vi "M-227 Stage Engine.vi"(0 "Unique Notifier Name":string="LevelStage", 11 "COM Port":string[](array[string])) -> ()   [LabVIEW 2016]
uses:
  Stages Controls/Stage Focus Control.ctl
  Stages Controls/Stage Status.ctl
  Stages Controls/Stage Notifier Element.ctl
  Stages Controls/Stage Actions.ctl
  <vilib>/Instr/_visa.llb/VISA Configure Serial Port (Instr).vi
panel:
  out "Position":dbl[](array[numeric])
  in  "Axis":T1={"Axis 1"=TRUE, "Axis 2"=TRUE, "Axis 3"=TRUE}
  in  "ReInitialize":bool
  in  "Abort":bool
  in  "Velocity":dbl(ring)=0.05 items=["SUPER SLOW"=0.01, "SLOW"=0.05, "MEDIUM"=0.1, "FAST"=0.8]
  out "Status":T2
  in  "QUIT":bool
  in  "Focus Control":T3
  # "Left near"
  # "Left far"
  # "Right"
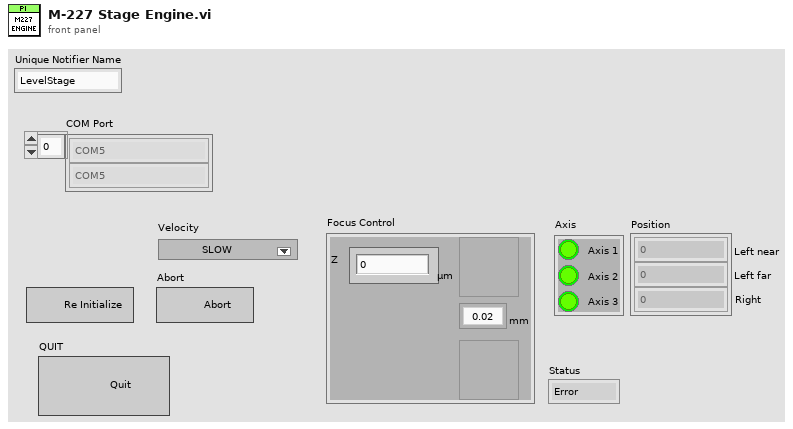
[diagram p1: front panel]
types:
  T1 = cluster{"Axis 1":bool, "Axis 2":bool, "Axis 3":bool}
  T2 = typedef "Stage Status.ctl" = enum16{"Error", "Abort", "Busy", "On Target"}
  T3 = typedef "Stage Focus Control.ctl" = cluster{"Focus Step (um)":enum16{"0.02", "0.05", "0.1", "0.5", "1", "2", "5", "10", "20"}, "Focus Up":bool, "Focus Down":bool, "Z ":dbl}
  T4 = typedef "Stage Actions.ctl" = enum16{"Get Position", "MVR", "MOVE", "HALT", "ONTARGET", "ERROR", "REFERENCE", "INIT", "VELOCITY", "STATUS", "EXIT", "HOME", "ZEROPOS", "NANOPOS", "ANALOG", "QUIT"}
  T5 = typedef "Stage Notifier Element.ctl" = cluster{"Action":T4, "Axis":bool[], "Setpoint":dbl[], "Velocity":dbl, "Cmd Recvd?":bool, "Position":dbl[], "Status":T2, "Misc":variant}
  T6 = cluster{"Focus Step (um)":bool, "Focus Up":bool, "Focus Down":bool, "Z ":bool}
  T7 = enum16{"0.02", "0.05", "0.1", "0.5", "1", "2", "5", "10", "20"}
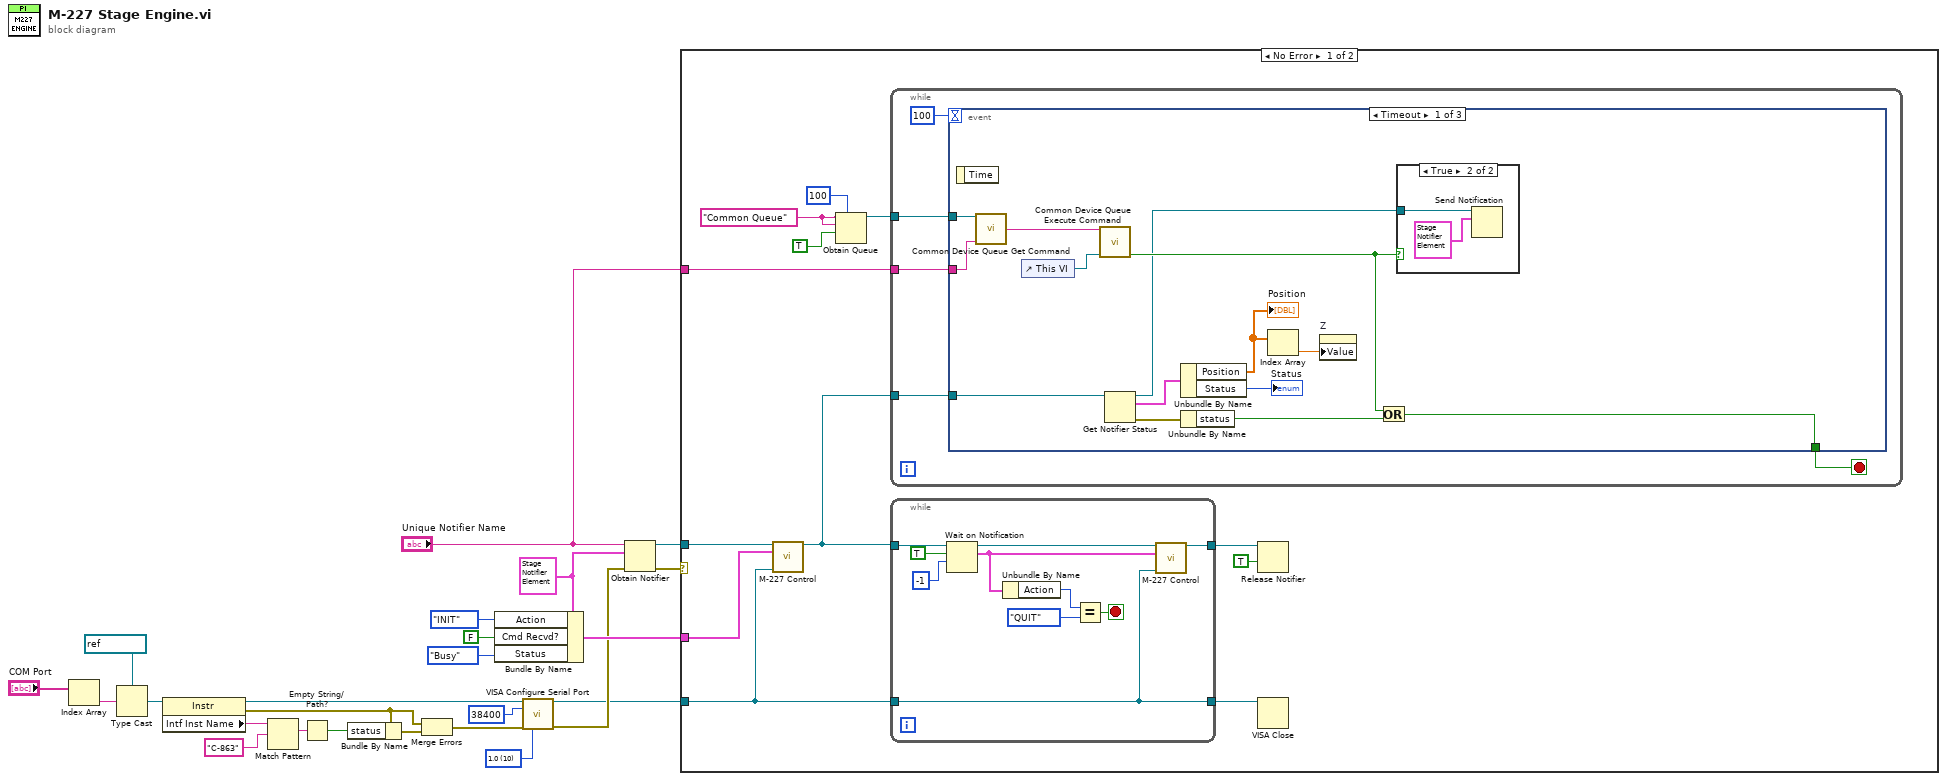
[diagram p0: block diagram]
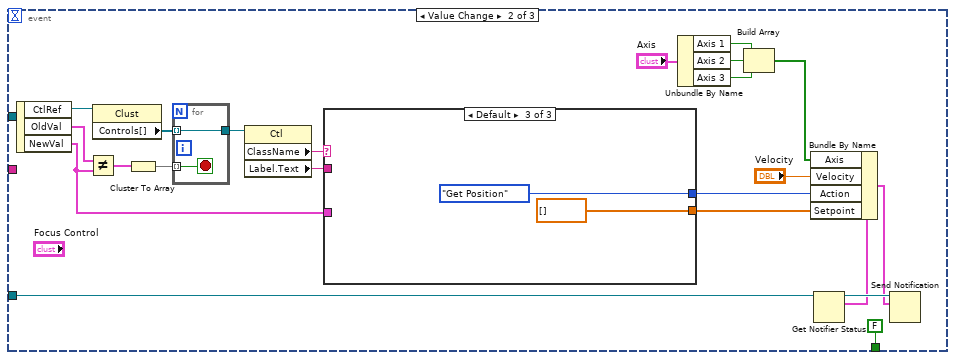
[diagram p3: hidden frame]
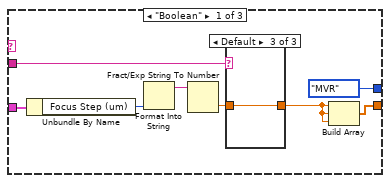
[diagram p4: hidden frame]
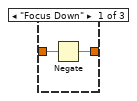
[diagram p5: hidden frame]
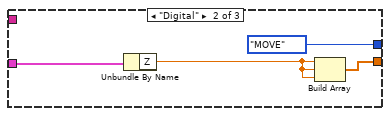
[diagram p7: hidden frame]
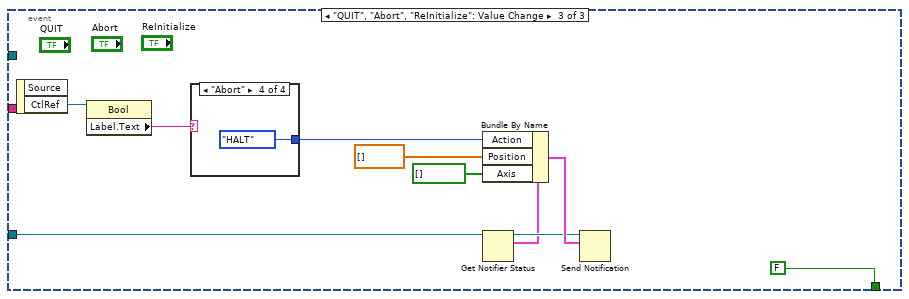
[diagram p8: hidden frame]
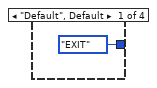
[diagram p9: hidden frame]
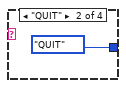
[diagram p10: hidden frame]
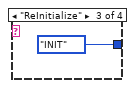
[diagram p11: hidden frame]
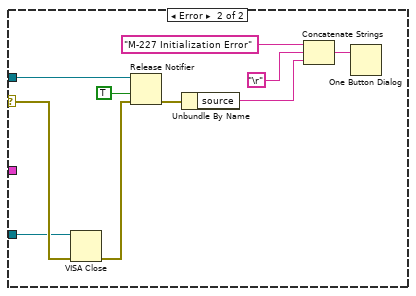
[diagram p12: hidden frame]
diagram:
  w7 = u16 10 items=["1.0"=10, "1.5"=15, "2.0"=20] ("stop bits (10: 1 bit)")
  w11 = T5 {"Action"=enum."Get Position", "Axis"=[], "Setpoint"=[], "Velocity"=0.5, "Cmd Recvd?"=FALSE, "Position"=[], "Status"=enum."Abort", "Misc"=variant} ("Stage Status")
  n1 = Index Array(array="COM Port") -> (element=w17:string)  [unwired: 1 in]
  n2 = Type Cast(type=refnum<visa-resource-name> "COM5" ("reference out"), x=w17) -> (*(type *) &x=w15:refnum<visa-resource-name>)
  n3 = property class="Instr"(reference=w15) -> (reference out=w4:refnum<visa-resource-name>, error out=w20:errorcluster, "Intf Inst Name"=w22:string)  [unwired: 1 in]
  n4 = Match Pattern(string=w22, regular expression="C-863") -> (match substring=w24:string)  [unwired: 1 in, 3 out]
  n5 = Empty String/Path?(string/path=w24) -> (empty?=w21:bool)
  n6 = Bundle By Name(cluster=w20, "status"=w21) -> (w19:errorcluster)
  n7 = Merge Errors(w20, w19) -> (w3:errorcluster)
  n8 = Bundle By Name(cluster=w11, "Action"=Stage_Actions."INIT", "Cmd Recvd?"=FALSE, "Status"=Stage_Status."Busy") -> (w9:T5)
  n9 = call-poly "VISA Configure Serial Port"("VISA resource name"=w4, "baud rate (9600)"=u32 38400, "error in (no error)"=w3, "stop bits (10: 1 bit)"=w7) -> ("VISA resource name out"=w2:refnum<visa-resource-name>, "error out"=w6:errorcluster)  [unwired: 10 in]
  n10 = Obtain Notifier(name (unnamed)="Unique Notifier Name", notification data type=w11, error in (no error)=w6) -> (notifier out=w1:refnum<notifier>, error out=w10:errorcluster)  [unwired: 1 in, 1 out]
  n11 = case shown="No Error" w10 {
    selector: w10 -> [_ w125]
    tunnel: w2 -> [w27 w124]
    tunnel: w9 -> [w28 _]
    tunnel: "Unique Notifier Name" -> [w31 _]
    tunnel: w1 -> [w30 w126]
    frame No Error {
      w33 = "Common Queue" ("Unique Notifier Name")
      n12 = call "M-227 Control.vi"("M-227 Notifier"=w30, "Stage Action"=w28, "VISA In"=w27) -> ("M-227 Notifier (Dup)"=w29:refnum<notifier>)  [unwired: 12 in]
      n13 = Obtain Queue(max queue size (-1, unlimited)=100, name (unnamed)=w33, element data type=w33, create if not found? (T)=TRUE) -> (queue out=w32:refnum<queue>)  [unwired: 1 in, 2 out]
      n14 = while {
        tunnel: w29 -> [w49]
        tunnel: w32 -> [w48]
        tunnel: w31 -> [w47]
        stop <- w50 stop-if-true
        n15 = event shown="[0] Timeout" {
          selector: _ -> [_ _ _]
          dyn-events: _ -> [_ _ _]
          timeout: 100 -> [_ _ _]
          tunnel: [w54 FALSE ("status") FALSE ("status")] -> w50
          tunnel: w49 -> [w64 w78 w115]
          tunnel: w48 -> [w57 _ _]
          tunnel: w47 -> [w56 _ _]
          event Timeout {
            n16 = event-data() -> ()  [unwired: 1 in, 1 out]
            n17 = call "Common Device Queue Get Command.vi"("Common Queue"=w57, "Notifier Name"=w56) -> ("Command"=w59:string)  [unwired: 12 in, 1 out]
            n18 = control-ref of="This VI"() -> (w58:refnum<vi>)
            n19 = call "Common Device Queue Execute Command.vi"("Common Command"=w59, "VI Refnum"=w58) -> ("Quit?"=w53:bool)  [unwired: 12 in, 1 out]
            n20 = Get Notifier Status(notifier=w64) -> (notifier out=w52:refnum<notifier>, current notification=w63:T5, error out=w61:errorcluster)  [unwired: 1 in, 2 out]
            n21 = Unbundle By Name(w63) -> ("Position"=w62:dbl[], "Status"=→"Status":T2)
            "Position" <- w62
            n22 = Unbundle By Name(w61) -> ("status"=w55:bool)
            n23 = Index Array(array=w62) -> (element=w65:dbl)  [unwired: 1 in]
            n24 = property on="Z" class="DigNum (strict)"("Value"=w65) -> ()  [unwired: 2 in, 2 out]
            n25 = Or(x=w53, y=w55) -> (x .or. y?=w54:bool)
            n26 = case shown="True" w53 {
              tunnel: w52 -> [_ w67]
              frame False {
              }
              frame True {
                n27 = Send Notification(notification=T5 {"Action"=enum."QUIT", "Axis"=[], "Setpoint"=[], "Velocity"=0.5, "Cmd Recvd?"=FALSE, "Position"=[], "Status"=enum."Error", "Misc"=variant} ("Stage Status"), notifier=w67) -> ()  [unwired: 1 in, 2 out]
              }
            }
          }
          event Value Change {
            n28 = event-data() -> ("CtlRef"=w88:refnum<vi>, "OldVal"=w89:T3, "NewVal"=w82:T3)  [unwired: 1 in]
            n29 = Not Equal?(x=w89, y=w82) -> (x != y?=w87:T6)
            n30 = property class="Clust"(reference=w88) -> ("Controls[]"=w85:refnum<vi>[])  [unwired: 1 in, 2 out]
            n31 = Cluster To Array(cluster=w87) -> (array=w86:bool[])
            n32 = for {
              tunnel: w86 -> [w109] mode=indexing
              tunnel: [w108] -> w84
              tunnel: w85 -> [w108] mode=indexing
              stop <- w109 stop-if-true
            }
            n33 = property class="Ctl"(reference=w84) -> ("ClassName"=w83:string, "Label.Text"=w81:string)  [unwired: 1 in, 2 out]
            n34 = case shown="Default" w83 {
              tunnel: w82 -> [w96 w105 _]
              tunnel: w81 -> [w97 _ _]
              tunnel: [w92 w104 dbl[] []] -> w80
              tunnel: [Stage_Actions."MVR" ("Action") Stage_Actions."MOVE" ("Action") Stage_Actions."Get Position" ("Action")] -> w77
              frame "Boolean" {
                n35 = Unbundle By Name(w96) -> ("Focus Step (um)"=w94:T7)
                n36 = Format Into String(w94) -> (resulting string=w95:string)  [unwired: 3 in, 1 out]
                n37 = Fract/Exp String To Number(string=w95) -> (number=w93:dbl)  [unwired: 3 in, 1 out]
                n38 = case shown="Default" w97 {
                  tunnel: w93 -> [w99 w100 w101]
                  tunnel: [w98 w100 w101] -> w90
                  frame "Focus Down" {
                    n39 = Negate(x=w99) -> (-x=w98:dbl)
                  }
                  frame "Focus Up" {
                  }
                  frame Default {
                  }
                }
                n40 = Build Array(w90, w90, w90) -> (w92:dbl[])
              }
              frame "Digital" {
                n41 = Unbundle By Name(w105) -> ("Z"=w102:dbl)
                n42 = Build Array(w102, w102, w102) -> (w104:dbl[])
              }
              frame Default {
              }
            }
            n43 = Unbundle By Name("Axis") -> ("Axis 1"=w70:bool, "Axis 2"=w71:bool, "Axis 3"=w69:bool)
            n44 = Build Array(w70, w71, w69) -> (w68:bool[])
            n45 = Get Notifier Status(notifier=w78) -> (notifier out=w76:refnum<notifier>, current notification=w75:T5)  [unwired: 1 in, 3 out]
            n46 = Bundle By Name(cluster=w75, "Axis"=w68, "Velocity"="Velocity", "Action"=w77, "Setpoint"=w80) -> (w74:T5)
            n47 = Send Notification(notification=w74, notifier=w76) -> ()  [unwired: 1 in, 2 out]
          }
          event "QUIT", "Abort", "ReInitialize": Value Change {
            n48 = event-data() -> ("CtlRef"=w112:refnum<vi>)  [unwired: 1 in, 1 out]
            n49 = property class="Bool"(reference=w112) -> ("Label.Text"=w111:string)  [unwired: 1 in, 2 out]
            n50 = case shown="\"Abort\"" w111 {
              tunnel: [Stage_Actions."EXIT" ("Action") Stage_Actions."QUIT" ("Action") Stage_Actions."INIT" ("Action") Stage_Actions."HALT" ("Action")] -> w110
              frame "Default", Default {
              }
              frame "QUIT" {
              }
              frame "ReInitialize" {
              }
              frame "Abort" {
              }
            }
            n51 = Get Notifier Status(notifier=w115) -> (notifier out=w114:refnum<notifier>, current notification=w113:T5)  [unwired: 1 in, 3 out]
            n52 = Bundle By Name(cluster=w113, "Action"=w110, "Position"=dbl[] [], "Axis"=bool[] []) -> (w116:T5)
            n53 = Send Notification(notification=w116, notifier=w114) -> ()  [unwired: 1 in, 2 out]
          }
        }
      }
      n54 = while {
        tunnel: w29 -> [w44]
        tunnel: w27 -> [w37]
        tunnel: [w39] -> w26
        tunnel: [w37] -> w25
        stop <- w46 stop-if-true
        n55 = Wait on Notification(notifier=w44, ignore previous (F)=TRUE, timeout in ms (-1)=-1) -> (notifier out=w40:refnum<notifier>, notification=w38:T5)  [unwired: 1 in, 2 out]
        n56 = Unbundle By Name(w38) -> ("Action"=w42:T4)
        n57 = Equal?(x=w42, y=Stage_Actions."QUIT") -> (x = y?=w46:bool)
        n58 = call "M-227 Control.vi"("M-227 Notifier"=w40, "Stage Action"=w38, "VISA In"=w37) -> ("M-227 Notifier (Dup)"=w39:refnum<notifier>)  [unwired: 12 in]
      }
      n59 = Release Notifier(notifier=w26, force destroy? (F)=TRUE) -> ()  [unwired: 1 in, 3 out]
      n60 = VISA Close(VISA resource name=w25) -> ()  [unwired: 1 in, 1 out]
    }
    frame Error {
      n61 = VISA Close(VISA resource name=w124, error in (no error)=w125) -> (error out=w127:errorcluster)
      n62 = Release Notifier(notifier=w126, force destroy? (F)=TRUE, error in (no error)=w127) -> (error out=w132:errorcluster)  [unwired: 2 out]
      n63 = Unbundle By Name(w132) -> ("source"=w129:string)
      n64 = Concatenate Strings("M-227 Initialization Error", "\r", w129) -> (w128:string)
      n65 = One Button Dialog(message=w128) -> ()  [unwired: 1 in, 1 out]
    }
  }
